vi "High Speed Stream.vi"() -> ()   [LabVIEW 2023]
doc: "This VI demonstrates basic use of the High Speed Stream channel, a channel wire that communicates data between two parallel loops with efficiency nearly equal to the built-in Queue functions, but easily handling many of the complex scenarios for managing the lifetime of that connection."
uses:
  <vilib>/ChannelSupport/Channel Abort Instructions.ctl
  <extravilib>/ChannelInstances/High Speed Stream-i32/Abort Signal/Abort Signal.lvclass/Abort Signal.ctl
  <extravilib>/ChannelInstances/High Speed Stream-i32/_Read For Replicate.vi
  <extravilib>/ChannelInstances/High Speed Stream-i32/Instantiate.vi
  <extravilib>/ChannelInstances/High Speed Stream-i32/)Channel.vi
  <extravilib>/ChannelInstances/High Speed Stream-i32/Abort Signal/Init Signal.vi
  <extravilib>/ChannelInstances/High Speed Stream-i32.lvlib
  <extravilib>/ChannelInstances/High Speed Stream-i32/Abort Signal/Abort Signal.lvclass
panel:
  in  "Consumer Stop Value":i32=-1
  in  "Emergency Stop Producer":bool
  out "Data Consumed":i32(graph)
  out "Data Produced":i32(graph)
  in  "Stop Consumer":bool
  in  "Stop Producer":bool
  # "Overview: Demonstrates how to use the High Speed Stream, which is one of the channel wire templates that ships with LabVIEW. Streams are restricted to a single writer and a single reader to provide point-to-point communication. The High Speed Stream provides control for a wide variation in communication needs while maintaining performance that is nearly as good as the raw use of queue refnums. This example shows how signals raised from different parts of the program can be easily transmitted to the rest of the application. \nInstructions:\n1. Run the VI. Press the Normal Stop Producer button to see the producer stop and the consumer continue until it catches up. This is a normal stop generated from the producer.\n2. Run the VI again. Press the Emergency Stop Producer button to see both stop at the same time. This is an emergency stop generated from the producer.\n3. Run the VI again. Press the Stop Consumer button to see both stop at the same time. This is a pre-data-read stop generated from the consumer.\n4. Run the VI again. Change the Consumer Stop Value to a value between 0 and 9 to see both loops stop as soon as the consumer receives that value. This is a post-data-read stop generated from the consumer."
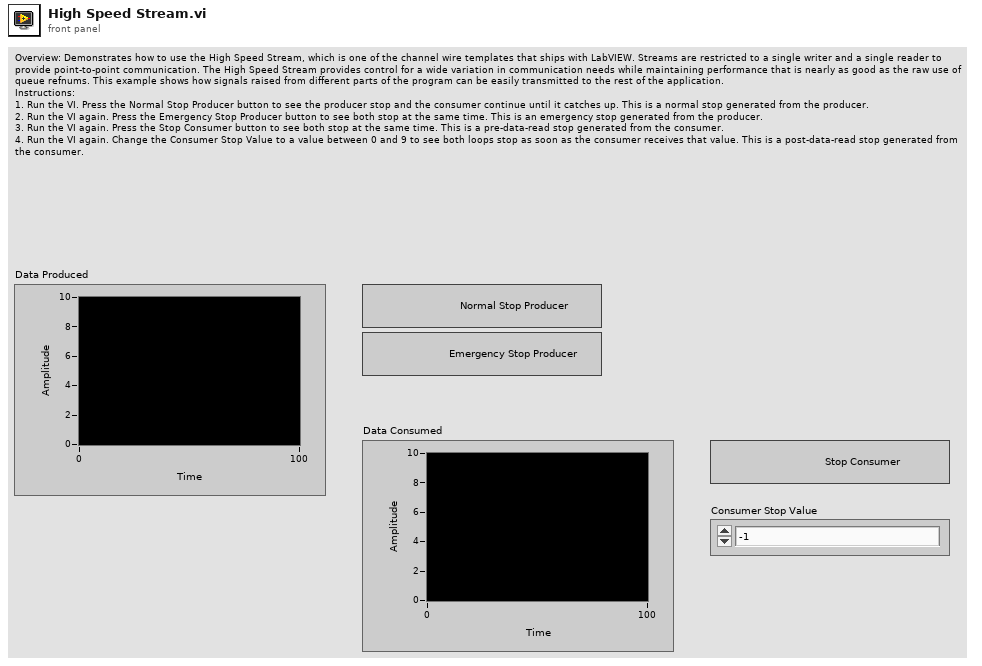
[diagram p1: front panel]
types:
  T1 = typedef "Channel Abort Instructions.ctl" = enum16{"No abort", "Abort now", "Abort if timeout"}
  T2 = typedef "High Speed Stream-i32.lvlib/)Channel.ctl" = refnum<queue>
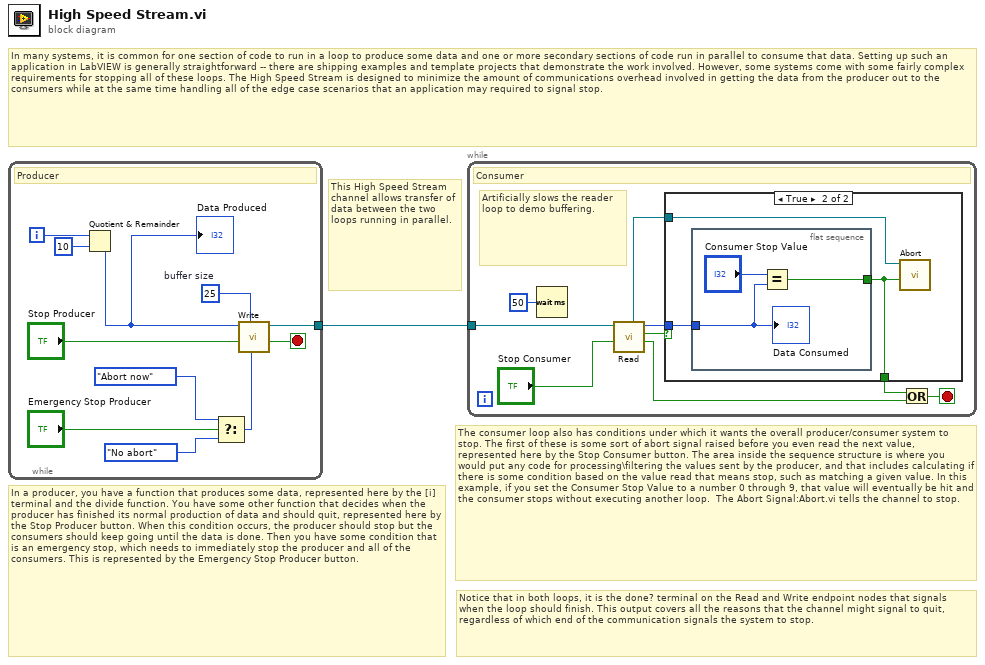
[diagram p0: block diagram]
diagram:
  # "Notice that in both loops, it is the done? terminal on the Read and Write endpoint nodes that signals when the loop should finish. This output covers all the reasons that the channel might signal to quit, regardless of which end of the communication signals the system to stop."
  # "The consumer loop also has conditions under which it wants the overall producer/consumer system to stop. The first of these is some sort of abort signal raised before you even read the next value, represented here by the Stop Consumer button. The area inside the sequence structure is where you would put any code for processing\\filtering the values sent by the producer, and that includes calculating if there is some condition based on the value read that means stop, such as matching a given value. In this example, if you set the Consumer Stop Value to a number 0 through 9, that value will eventually be hit and the consumer stops without executing another loop.  The Abort Signal:Abort.vi tells the channel to stop."
  # "This High Speed Stream channel allows transfer of data between the two loops running in parallel."
  # "In a producer, you have a function that produces some data, represented here by the [i] terminal and the divide function. You have some other function that decides when the producer has finished its normal production of data and should quit, represented here by the Stop Producer button. When this condition occurs, the producer should stop but the consumers should keep going until the data is done. Then you have some condition that is an emergency stop, which needs to immediately stop the producer and all of the consumers. This is represented by the Emergency Stop Producer button."
  # "In many systems, it is common for one section of code to run in a loop to produce some data and one or more secondary sections of code run in parallel to consume that data. Setting up such an application in LabVIEW is generally straightforward -- there are shipping examples and template projects that demonstrate the work involved. However, some systems come with some fairly complex requirements for stopping all of these loops. The High Speed Stream is designed to minimize the amount of communications overhead involved in getting the data from the producer out to the consumers while at the same time handling all of the edge case scenarios that an application may required to signal stop."
  n1 = while {
    tunnel: [w5] -> w1
    i -> [w8]
    stop <- w4 stop-if-true
    w6 = 25  # buffer size
    # "Producer"
    n2 = Quotient & Remainder(x=w8, y=10) -> (x-y*floor(x/y)=w7:i32)  [unwired: 1 out]
    "Data Produced" <- w7
    n3 = Select(t=Channel_Abort_Instructions."Abort now" ("abort instructions (no abort)"), s="Emergency Stop Producer", f=Channel_Abort_Instructions."No abort" ("abort instructions (no abort)")) -> (s? t:f=w3:T1)
    n4 = call <extravilib>:"Write.vi"("abort status (no abort)"=w3, "size (unlimited)"=w6, "last element? (F)"="Stop Producer", "element"=w7) -> ("done?"=w4:bool, "channel"=w5:T2)  [unwired: 5 in, 1 out]
  }
  n5 = while {
    tunnel: w1 -> [w18]
    stop <- w21 stop-if-true
    # "Artificially slows the reader loop to demo buffering."
    # "Consumer"
    n6 = Wait (ms)(milliseconds to wait=u32 50) -> ()  [unwired: 1 out]
    n7 = call <extravilib>:"Read.vi"("abort before read? (F)"="Stop Consumer", "channel"=w18) -> ("done?"=w14:bool, "element valid?"=w15:bool, "element"=w16:i32, "abort signal"=w17:refnum<class "Abort Signal.lvclass">)  [unwired: 5 in, 1 out]
    n8 = case shown="True" w15 {
      tunnel: w17 -> [_ w23]
      tunnel: w16 -> [_ w24]
      tunnel: [_ w22] -> w20
      frame False {
      }
      frame True {
        n9 = flat-sequence {
          tunnel: w24 -> [w26]
          tunnel: [w25] -> w22
          frame #0 {
            n10 = Equal?(x="Consumer Stop Value", y=w26) -> (x = y?=w25:bool)
            "Data Consumed" <- w26
          }
        }
        n11 = call <extravilib>:"Abort.vi"("abort? (T)"=w22, "abort signal"=w23) -> ()  [unwired: 9 in, 1 out]
      }
    }
    n12 = Or(x=w20, y=w14) -> (x .or. y?=w21:bool)
  }
